vi "Test CNV Algo and graph single instance.vi"() -> ()   [LabVIEW 2019]
uses:
  <vilib>/Analysis/3filter.llb/Filter Passband Type.ctl
  <vilib>/Analysis/baseanly.llb/Mean (DBL).vi
  <vilib>/Utility/file.llb/Read Delimited Spreadsheet (DBL).vi
  <userlib>/_OpenG.lib/array/array.llb/Search 1D Array (DBL)__ogtk.vi
  <vilib>/Analysis/3filter.llb/Butterworth Filter (DBL).vi
  <vilib>/Analysis/NI_AALBase.lvlib
  <vilib>/ptbypt/NI_PtbyPt.lvlib
panel:
  out "slope":dbl(graph)
  out "process 1":dbl(graph)
  out "Numeric":i32
  out "analyzed signal":dbl[](graph)
  out "segmented graph":dbl[](graph)
  in  "Next Button":bool
  in  "stop show":bool
  out "Indices of Elements":i32[](array[numeric])
  out "data filt":dbl(graph)
  out "mean":dbl format="%0.2f"
  out "error":i32
  out "Waveform Graph Filtered":dbl[](graph)
  out "Waveform Graph":dbl[](graph)
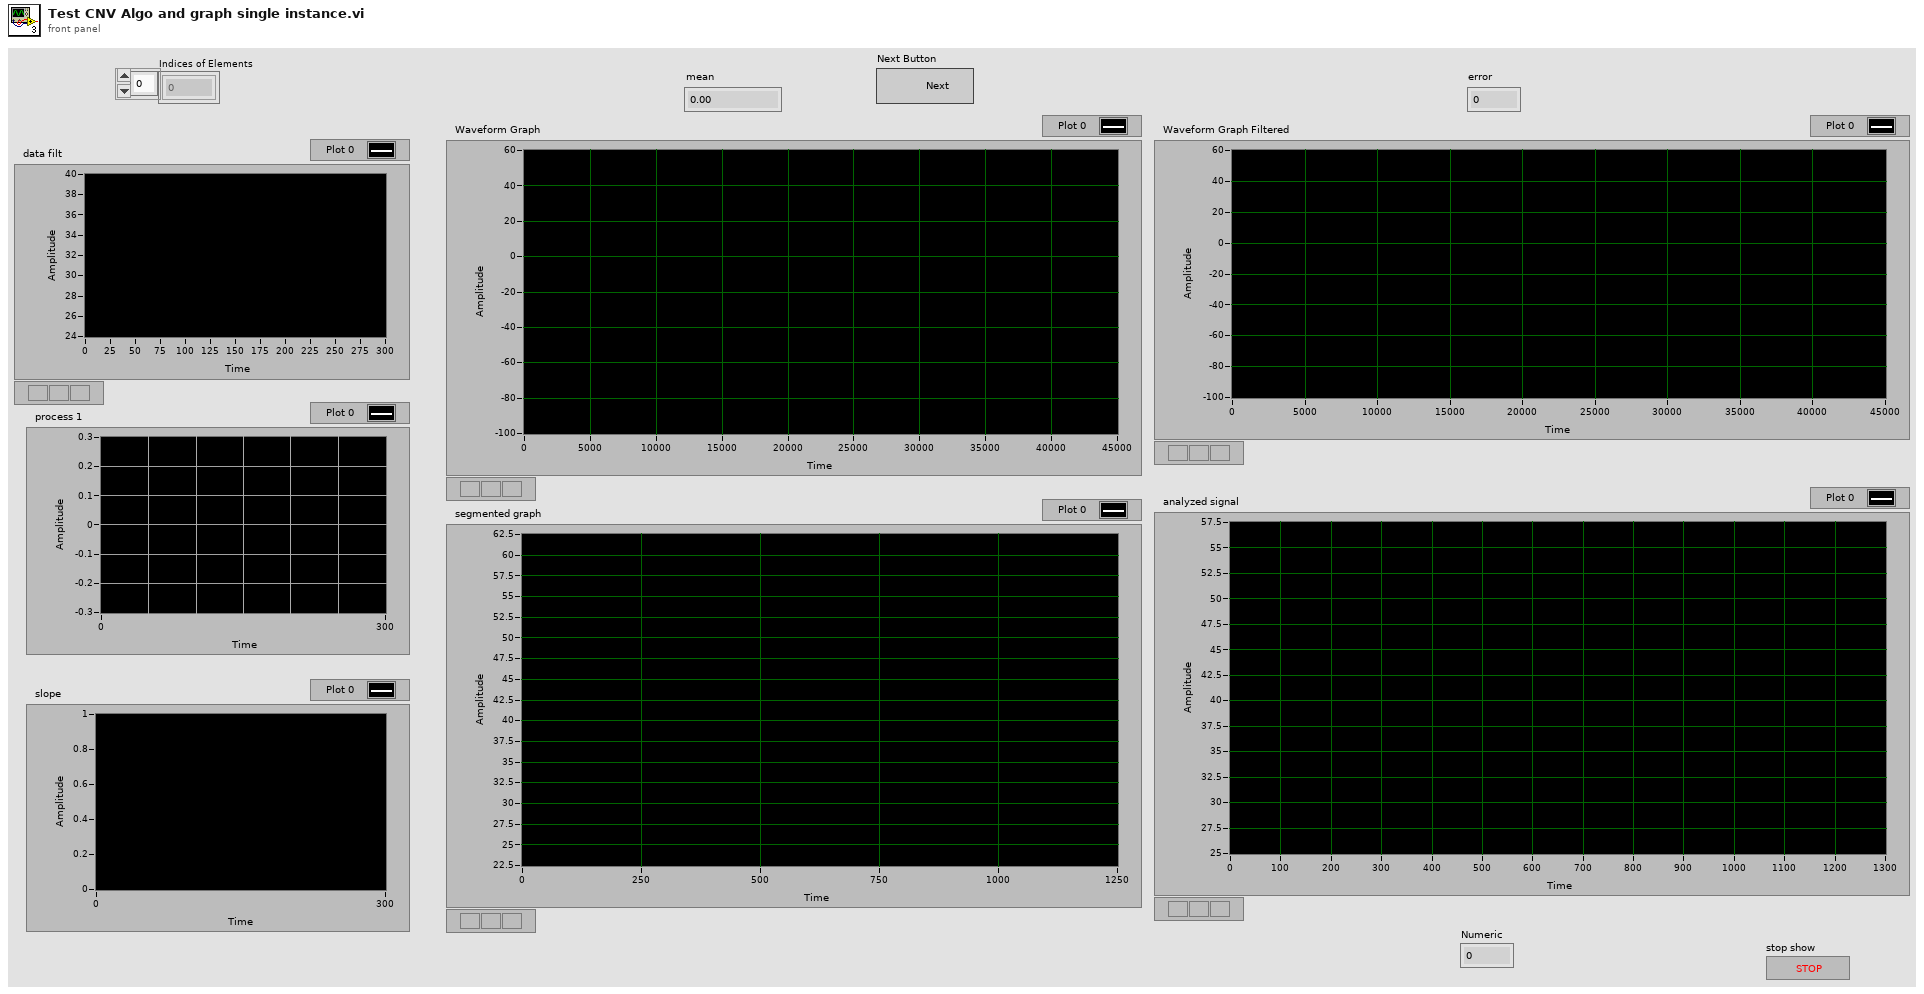
[diagram p1: front panel]
types:
  T1 = typedef "NI_AALBase.lvlib/Filter Passband Type.ctl" = enum32{"Lowpass", "Highpass", "Bandpass", "Bandstop"}
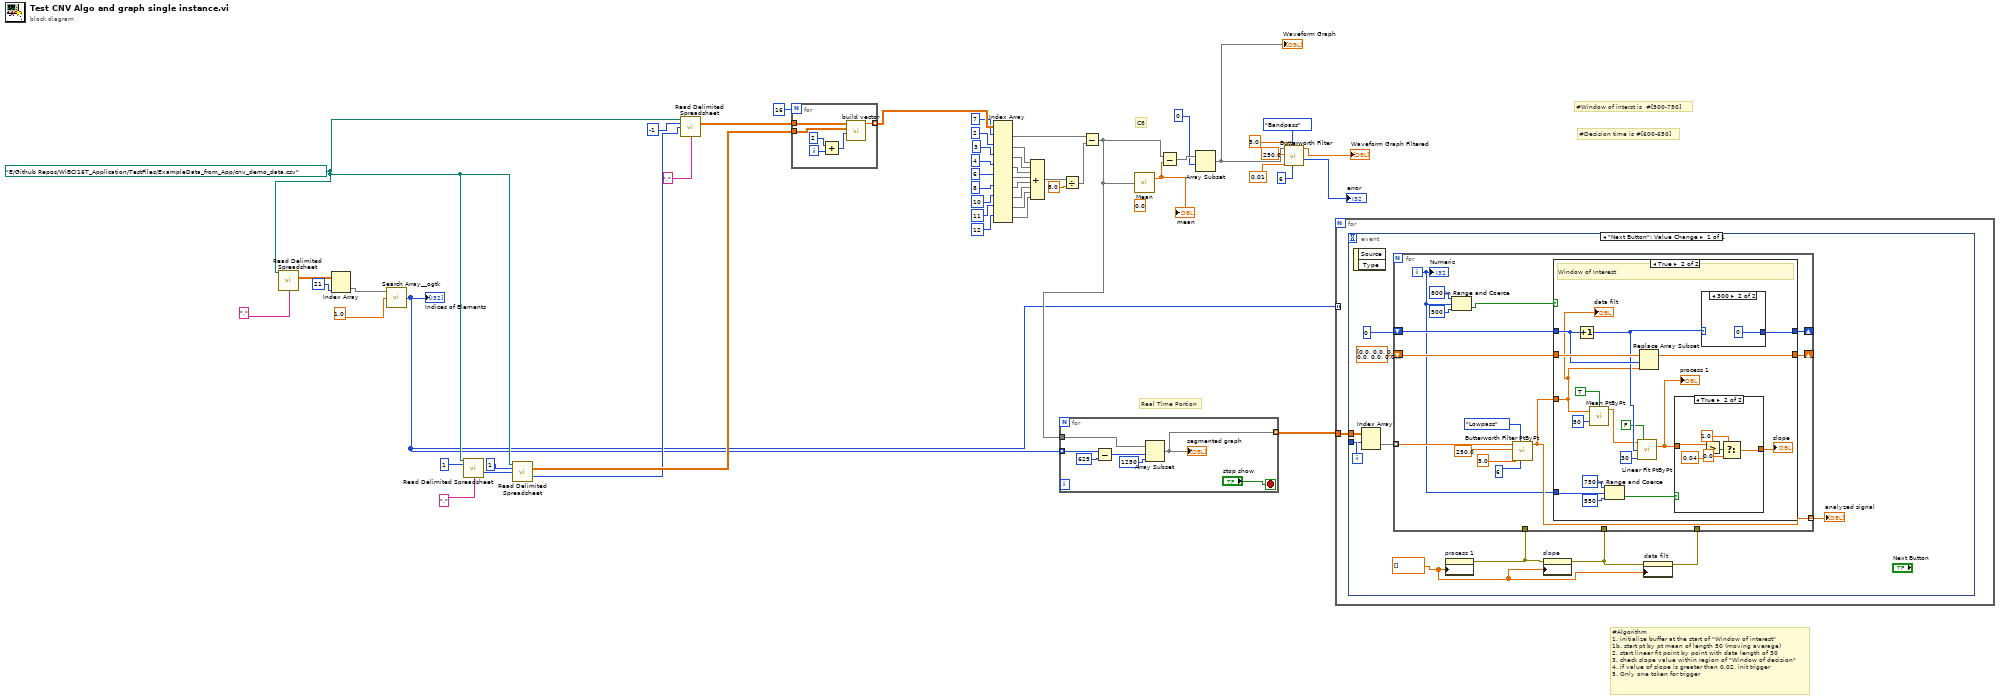
[diagram p0: block diagram]
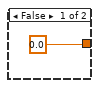
[diagram p3: hidden frame]
diagram:
  (unwired) 0.0
  w13 = path "E:/Github Repos/WiBCI16T_Application/TestFiles/ExampleData_from_App/cnv_demo_data.csv" ("file path (dialog if empty)")
  # "#Algorithm\n1. initialize buffer at the start of \"Window of interest\"\n1b. start pt by pt mean of length 50 (moving average)\n2. start linear fit point by point with data length of 30\n3. check slope value within region of \"Window of decision\"\n4. if value of slope is greater than 0.02, init trigger\n5. Only one token for trigger"
  # "#Decision time is #[600-650]"
  # "#Window of interst is  #[500-750]"
  # "Real Time Portion"
  # "C8"
  n1 = call-poly <vilib>:"Read Delimited Spreadsheet.vi"("file path (dialog if empty)"=w13, "delimiter (\\t)"=",") -> ("all rows"=w17:dbl[][])  [unwired: 8 in, 5 out]
  n2 = Index Array(array=w17, index (col)=21 ("disabled index (col)")) -> (element=w12:dbl[])  [unwired: 1 in]
  n3 = call-poly <userlib>:"Search Array__ogtk.vi"("Array"=w12, "Element Data"=1.0 ("element")) -> ("Indices of Elements"=w1:i32[])  [unwired: 7 in]
  "Indices of Elements" <- w1
  n4 = call-poly <vilib>:"Read Delimited Spreadsheet.vi"("file path (dialog if empty)"=w13, "number of rows (all:-1)"=1, "delimiter (\\t)"=",") -> ("mark after read (chars.)"=w50:i32)  [unwired: 7 in, 5 out]
  n5 = call-poly <vilib>:"Read Delimited Spreadsheet.vi"("file path (dialog if empty)"=w13, "number of rows (all:-1)"=1, "start of read offset (chars.:0)"=w50) -> ("all rows"=w48:dbl[][], "mark after read (chars.)"=w4:i32)  [unwired: 7 in, 4 out]
  n6 = call-poly <vilib>:"Read Delimited Spreadsheet.vi"("file path (dialog if empty)"=w13, "number of rows (all:-1)"=-1, "start of read offset (chars.:0)"=w4, "delimiter (\\t)"=",") -> ("all rows"=w24:dbl[][])  [unwired: 6 in, 5 out]
  n7 = for {
    N: 16 -> [_]
    tunnel: w24 -> [w58]
    tunnel: w48 -> [w57]
    tunnel: [w53] -> w46 mode=indexing
    i -> [w56]
    n8 = Add(x=2, y=w56) -> (x+y=w54:i32)
    n9 = call "build vector.vi"("Index"=w54, "first element"=w57, "diff data"=w58) -> ("Rebuild Vector"=w53:dbl[])  [unwired: 8 in]
  }
  n10 = Index Array(array=w46, index (row) #1=7 ("disabled index (col)"), index (row) #2=2 ("index (row)"), index (row) #3=3 ("index (row)"), index (row) #4=4 ("index (row)"), index (row) #5=6 ("index (row)"), index (row) #6=8 ("index (row)"), index (row) #7=10 ("index (row)"), index (row) #8=11 ("index (row)"), index (row) #9=12 ("index (row)")) -> (element #1=w26:dbl[], element #2=w36:dbl[], element #3=w35:dbl[], element #4=w34:dbl[], element #5=w33:dbl[], element #6=w32:dbl[], element #7=w31:dbl[], element #8=w30:dbl[], element #9=w29:dbl[])  [unwired: 9 in]
  n11 = Compound Arithmetic op=ADD(w36, w35, w34, w33, w32, w31, w30, w29) -> (w28:dbl[])
  n12 = Divide(x=w28, y=8.0) -> (x/y=w25:dbl[])
  n13 = Subtract(x=w26, y=w25) -> (x-y=w3:dbl[])
  n14 = for {
    tunnel: w1 -> [w64] mode=indexing
    tunnel: w3 -> [w65]
    tunnel: [w59] -> w2 mode=indexing
    stop <- "stop show" stop-if-true
    n15 = Subtract(x=w64, y=625) -> (x-y=w61:i32)
    n16 = Array Subset(array=w65, index=w61, length=1250) -> (w59:dbl[])
    "segmented graph" <- w59
  }
  n17 = call-poly <vilib>:"Mean.vi"("X"=w3) -> ("mean"=w14:dbl)  [unwired: 1 out]
  "mean" <- w14
  n18 = Subtract(x=w3, y=w14) -> (x-y=w8:dbl[])
  n19 = Array Subset(array=w8, index=0) -> (w6:dbl[])  [unwired: 1 in]
  "Waveform Graph" <- w6
  n20 = call-poly <vilib>:"Butterworth Filter.vi"("order"=6, "filter type"=Filter_Passband_Type."Bandpass", "low cutoff freq: fl"=0.01, "high cutoff freq: fh"=5.0, "sampling freq: fs"=250.0, "X"=w6) -> ("error"=→"error":i32, "Filtered X"=→"Waveform Graph Filtered":dbl[])  [unwired: 2 in]
  n21 = for {
    tunnel: w2 -> [w67]
    tunnel: w1 -> [_] mode=indexing
    i -> [w66]
    n22 = event shown="[0] \"Next Button\": Value Change" {
      selector: _ -> [_]
      dyn-events: _ -> [_]
      timeout: _ -> [_]
      tunnel: w67 -> [w77]
      tunnel: w66 -> [w75]
      event "Next Button": Value Change {
        w69 = dbl[] []
        n23 = event-data() -> ()  [unwired: 1 in, 2 out]
        n24 = Index Array(array=w77, index (row)=w75) -> (element=w76:dbl[])  [unwired: 1 in]
        n25 = property on="process 1" class="WFChart (strict)"("History Data"=w69) -> (error out=w71:errorcluster)  [unwired: 2 in, 1 out]
        n26 = property on="slope" class="WFChart (strict)"(error in=w71, "History Data"=w69) -> (error out=w70:errorcluster)  [unwired: 1 in, 1 out]
        n27 = property on="data filt" class="WFChart (strict)"(error in=w70, "History Data"=w69) -> (error out=w68:errorcluster)  [unwired: 1 in, 1 out]
        n28 = for {
          tunnel: w76 -> [w87] mode=indexing
          tunnel: [w83] -> w74 mode=indexing
          shift-right: [w79] -> _
          shift-left: dbl[] [0.0, 0.0, 0.0, 0.0, 0.0, 0.0, 0.0, 0.0, 0.0, 0.0, 0.0, 0.0, 0.0, 0.0, 0.0, 0.0, 0.0, 0.0, 0.0, 0.0, 0.0, 0.0, 0.0, 0.0, 0.0, 0.0, 0.0, 0.0, 0.0, 0.0, 0.0, 0.0, 0.0, 0.0, 0.0, 0.0, 0.0, 0.0, 0.0, 0.0, 0.0, 0.0, 0.0, 0.0, 0.0, 0.0, 0.0, 0.0, 0.0, 0.0, 0.0, 0.0, 0.0, 0.0, 0.0, 0.0, 0.0, 0.0, 0.0, 0.0, 0.0, 0.0, 0.0, 0.0, 0.0, 0.0, 0.0, 0.0, 0.0, 0.0, 0.0, 0.0, 0.0, 0.0, 0.0, 0.0, 0.0, 0.0, 0.0, 0.0, 0.0, 0.0, 0.0, 0.0, 0.0, 0.0, 0.0, 0.0, 0.0, 0.0, 0.0, 0.0, 0.0, 0.0, 0.0, 0.0, 0.0, 0.0, 0.0, 0.0] -> [w82]
          shift-right: [w80] -> _
          shift-left: 0 -> [w81]
          tunnel: w71 -> [_]
          tunnel: w70 -> [_]
          tunnel: w68 -> [_]
          i -> [w78]
          n29 = In Range and Coerce(upper limit=800, x=w78, lower limit=500) -> (In Range?=w84:bool)  [unwired: 1 out]
          n30 = call <vilib>:"Butterworth Filter PtByPt.vi"("order"=6, "filter type"=Filter_Passband_Type."Lowpass", "low cutoff freq: fl"=5.0, "sampling freq: fs"=250.0, "x"=w87) -> ("Filtered x"=w83:dbl)  [unwired: 4 in, 1 out]
          n31 = case shown="True" w84 {
            tunnel: w83 -> [_ w95]
            tunnel: w82 -> [w92 w110]
            tunnel: w81 -> [w93 w109]
            tunnel: [w93 w108] -> w80
            tunnel: [w92 w107] -> w79
            tunnel: w78 -> [_ w102]
            frame False {
              # "Ignore"
            }
            frame True {
              # "Window of Interest"
              n32 = Increment(x=w109) -> (x+1=w105:i32)
              n33 = call <vilib>:"Mean PtByPt.vi"("x"=w95, "sample length"=50, "initialize"=TRUE) -> ("mean"=w96:dbl)  [unwired: 1 in, 1 out]
              n34 = In Range and Coerce(upper limit=750, x=w102, lower limit=550) -> (In Range?=w101:bool)  [unwired: 1 out]
              n35 = call <vilib>:"Linear Fit PtByPt.vi"("y"=w96, "initialize"=FALSE, "x"=w105, "sample length"=30) -> ("slope"=w94:dbl)  [unwired: 7 in, 4 out]
              "process 1" <- w94
              n36 = Replace Array Subset(array=w110, new element=w95, index=w109) -> (w107:dbl[])
              n37 = case shown="True" w101 {
                tunnel: w94 -> [_ w117]
                tunnel: [0.0 w112] -> w100
                frame False {
                }
                frame True {
                  n38 = Greater?(x=w117, y=0.04) -> (0:w115:bool)
                  n39 = Select(t=1.0, s=w115, f=0.0) -> (s? t:f=w112:dbl)
                }
              }
              "slope" <- w100
              n40 = case shown="300" w105 {
                selector: w105 -> [w118 _]
                tunnel: [w118 0] -> w108
                frame 0, Default {
                }
                frame 300 {
                }
              }
              "data filt" <- w95
            }
          }
          "Numeric" <- w78
        }
        "analyzed signal" <- w74
      }
    }
  }
